vi "读写颜色检测参数-INI.vi"(6 "T写入F读取":bool, 8 "error in (no error)":errorcluster, 10 "configuration file path":path, 11 "相机设置输入":T1) -> (0 "error out":errorcluster, 3 "相机设置输出":T1)   [LabVIEW 2018]
uses:
  <vilib>/Utility/config.llb/NI_LVConfig.lvlib
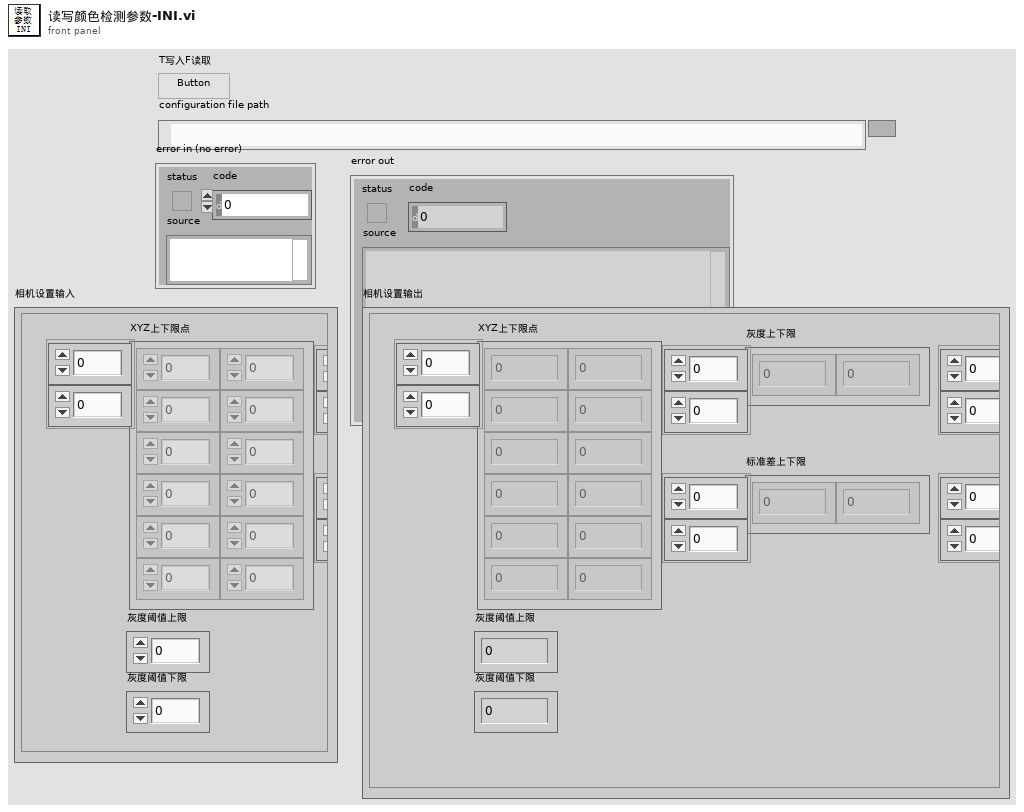
[diagram p1: front panel]
types:
  T1 = typedef "颜色检测参数ini.ctl" = cluster{"XYZ上下限点":dbl[][], "灰度上下限":dbl[][], "灰度上下限 2":dbl[][], "标准差上下限":dbl[][], "标准差上下限 2":dbl[][], "灰度阈值上限":dbl, "灰度阈值下限":dbl}
  T2 = typedef "NI_LVConfig.lvlib/Config Data RefNum.ctl" = refnum<k1>
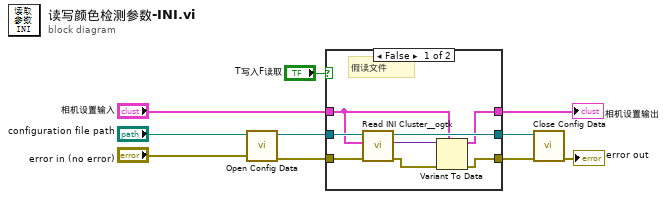
[diagram p0: block diagram]
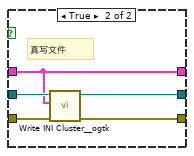
[diagram p2: hidden frame]
diagram:
  n1 = call <vilib>:"Open Config Data.vi"("error in (no error)"="error in (no error)", "configuration file path"="configuration file path") -> ("error out"=w9:errorcluster, "refnum"=w10:T2)  [unwired: 7 in, 1 out]
  n2 = case shown="False" "T写入F读取" {
    tunnel: w10 -> [w18 w23]
    tunnel: w9 -> [w17 w21]
    tunnel: [w16 w22] -> w8
    tunnel: [w13 w20] -> w7
    tunnel: "相机设置输入" -> [w12 w19]
    tunnel: [w11 w19] -> w1
    frame False {
      # "假读文件"
      n3 = call "Read INI Cluster__ogtk.vi"("error in (no error)"=w17, "INI Fomatted Cluster Type"=w12, "refnum"=w18) -> ("error out"=w14:errorcluster, "INI Fomatted Cluster"=w15:variant, "dup refnum"=w16:T2)  [unwired: 4 in, 2 out]
      n4 = Variant To Data(error in=w14, type=w12, Variant=w15) -> (data=w11:T1, error out=w13:errorcluster)
    }
    frame True {
      # "真写文件"
      n5 = call "Write INI Cluster__ogtk.vi"("error in (no error)"=w21, "INI Fomatted Cluster"=w19, "refnum"=w23) -> ("error out"=w20:errorcluster, "dup refnum"=w22:T2)  [unwired: 7 in]
    }
  }
  "相机设置输出" <- w1
  n6 = call <vilib>:"Close Config Data.vi"("error in (no error)"=w7, "refnum"=w8) -> ("error out"=→"error out":errorcluster)  [unwired: 8 in, 1 out]
